vi "计算输入字符串时间.vi"() -> ()   [LabVIEW 2018]
panel:
  out "时间(s)":dbl
  in  "确定按钮":bool
  in  "字符串":string
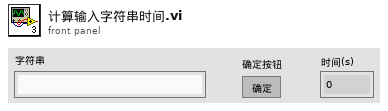
[diagram p1: front panel]
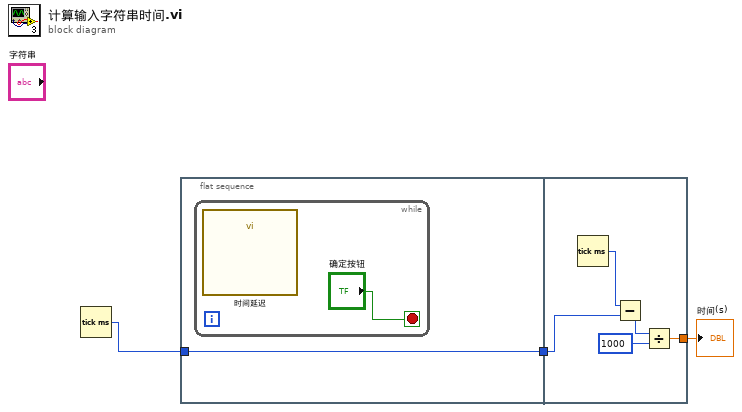
[diagram p0: block diagram]
diagram:
  n1 = Tick Count (ms)() -> (millisecond timer value=w2:u32)
  n2 = flat-sequence {
    tunnel: [w4] -> w3
    tunnel: w2 -> [w4]
    tunnel: w3 -> [w9]
    tunnel: [w6] -> w1
    frame #0 {
      n3 = while {
        stop <- "确定按钮" stop-if-true
        n4 = call "时间延迟"() -> ()  [unwired: 11 in, 1 out]
      }
    }
    frame #1 {
      n5 = Tick Count (ms)() -> (millisecond timer value=w10:u32)
      n6 = Subtract(x=w10, y=w9) -> (x-y=w8:u32)
      n7 = Divide(x=w8, y=u32 1000) -> (x/y=w6:dbl)
    }
  }
  "时间(s)" <- w1
